vi "Read termination character.vi"(8 "error in (no error)":errorcluster, 11 "Serial Comms in":refnum<class "Serial Comms.lvclass">) -> (0 "error out":errorcluster, 2 "Enable Termination Character":bool, 3 "Serial Comms out":refnum<class "Serial Comms.lvclass">)   [LabVIEW 2020, in "Generic_Comms.lvlib" / "Serial Comms.lvclass"]
uses:
  Serial Comms.lvclass
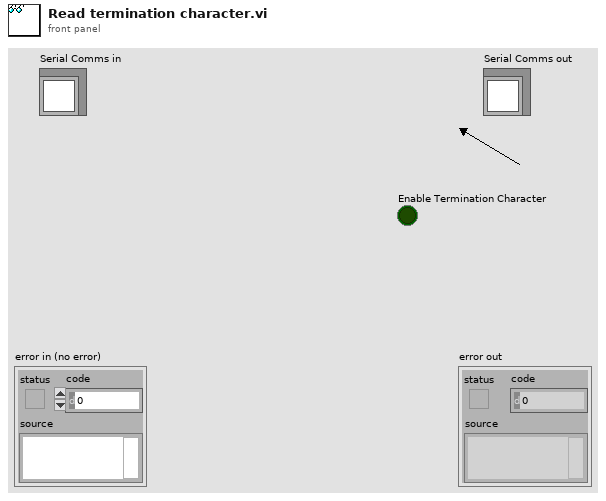
[diagram p1: front panel]
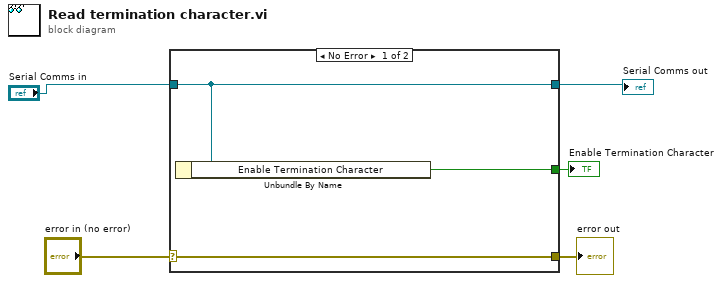
[diagram p0: block diagram]
diagram:
  n1 = case shown="No Error" "error in (no error)" {
    selector: "error in (no error)" -> [w8 w9]
    tunnel: [w8 w9] -> w4
    tunnel: [w7 w10] -> w2
    tunnel: "Serial Comms in" -> [w7 w10]
    tunnel: [w6 _] -> w1
    frame No Error {
      n2 = Unbundle By Name(w7) -> ("Enable Termination Character"=w6:bool)
    }
    frame Error {
    }
  }
  "error out" <- w4
  "Serial Comms out" <- w2
  "Enable Termination Character" <- w1
